vi "DQMH_Event_DialogTest.vi"() -> ()   [LabVIEW 2016]
panel:
  in  "EventData":T1={"ModuleName"="TestStation.lvlib", "EventType"=enum."Request", "AddButtonInAPITester"=FALSE, "EventName"="MyRequest", "EventDescription"="Some Description"}
  out "Numeric Control":i32=3
  out "Array":string[][](array[string])=[["Module", "Ring", ""], ["Event Type", "Ring", "Request,Broadcast,Request and Wait for Reply,Round Trip (Request and Wait for Reply + Broadcast)"], ["Add Tester Button", "Boolean", ""], ["Enqueue Message VI", "RadioButtonsControl", ""], ["Existing Request", "Ring", ""], ["Custom Enqueue VI", "Path", ""], ["Broadcast Argument Source", "RadioButtonsControl", ""], ["Event Name", "String", ""], ["Round Trip (Broadcast)", "String", ""], ["Event Description", "String", ""], ["OK", "Boolean", ""], ["Cancel", "Boolean", ""], ["Help", "Boolean", ""], ["Round Trip (Request)", "String", ""], ["Step 6", "String", ""], ["Context Help", "Ring", "Request Event:\nAn event generated by a caller that the module is registered to receive. Typically a request event is a request for the module to \"Do something\".,Broadcast Event:\nAn event generated by the module to let any external code that is registered  to receive the event know that \"Something happened\".,Request and Wait for Reply:\nA request event where the event generator waits for the module to process the request and return the request processing results. This provides synchronous request and reply functionality.,Round Trip:\nA request and wait for reply event and a broadcast event where the reply payload data type is the same as the broadcast argument.,"]]
  out "NI.LV.Dialog Found":bool=TRUE
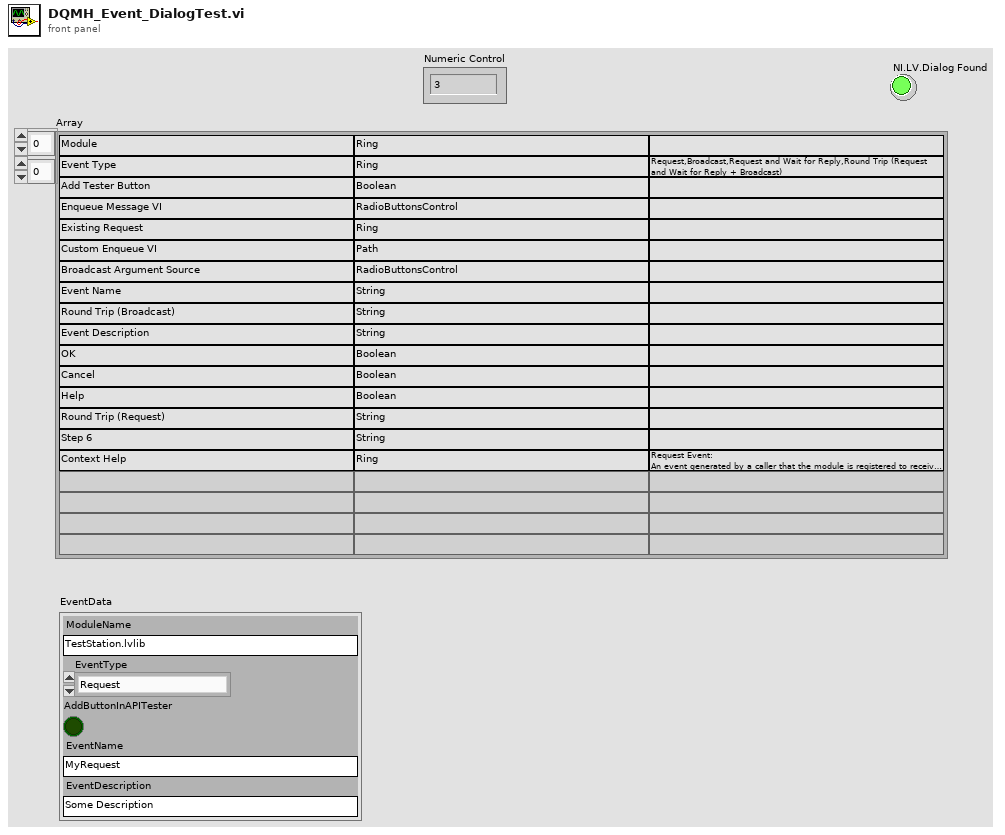
[diagram p1: front panel]
types:
  T1 = cluster{"ModuleName":string, "EventType":enum16{"Request", "Broadcast", "Request and Wait for Reply", "Round Trip"}, "AddButtonInAPITester":bool, "EventName":string, "EventDescription":string}
  T2 = enum32{"Bad", "Idle", "Run top level", "Running"}
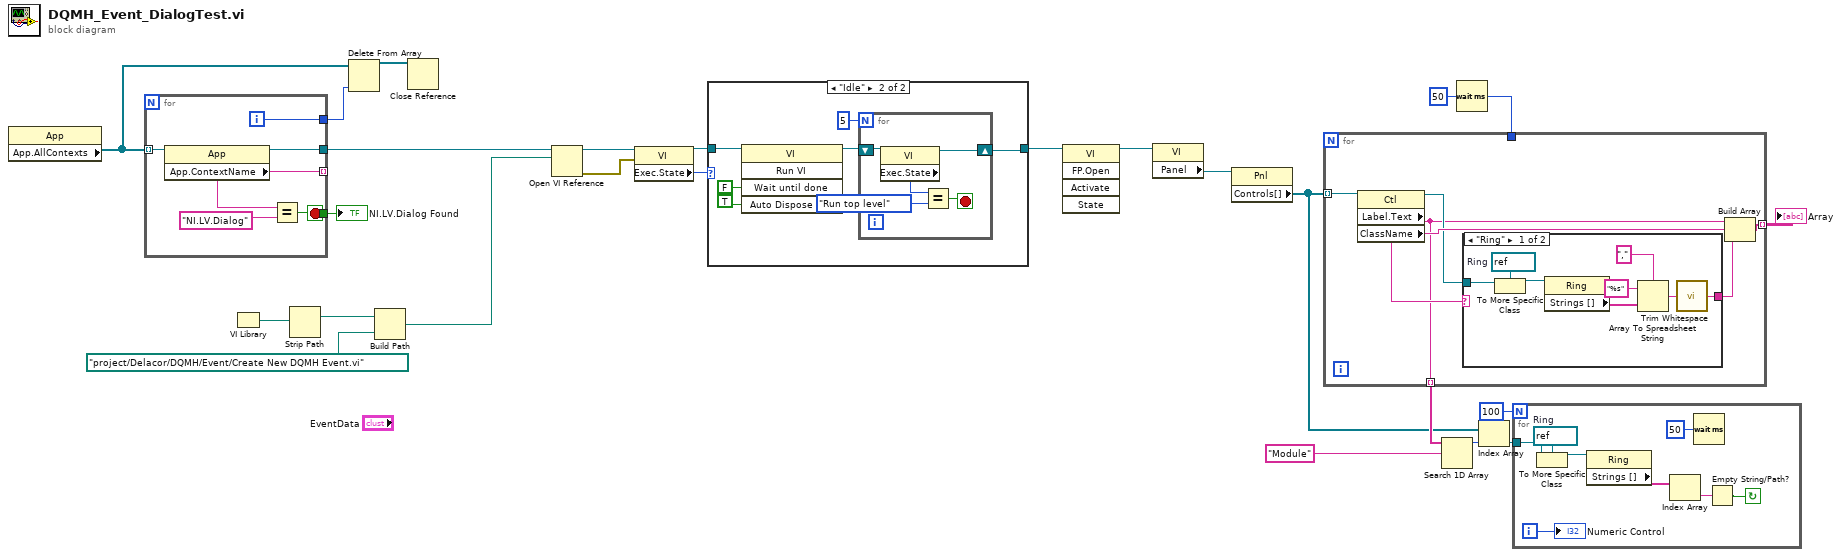
[diagram p0: block diagram]
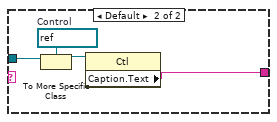
[diagram p2: hidden frame]
diagram:
  n1 = property class="App"() -> ("App.AllContexts"=w24:refnum<vi>[])  [unwired: 2 in, 2 out]
  n2 = for {
    tunnel: w24 -> [w31] mode=indexing
    tunnel: [w29] -> _ mode=indexing
    tunnel: [w28] -> w25
    tunnel: [w27] -> w23
    tunnel: [w26] -> w21
    i -> [w27]
    stop <- w28 stop-if-true
    n3 = property class="App"(reference=w31) -> (reference out=w26:refnum<vi>, "App.ContextName"=w29:string)  [unwired: 1 in, 1 out]
    n4 = Equal?(x=w29, y="NI.LV.Dialog" ("App.ContextName")) -> (x = y?=w28:bool)
  }
  "NI.LV.Dialog Found" <- w25
  n5 = VI Library() -> (path=w20:path)
  n6 = Strip Path(path=w20) -> (stripped path=w19:path)  [unwired: 1 out]
  n7 = Delete From Array(array=w24, index=w23) -> (array with subset deleted=w22:refnum<vi>[])  [unwired: 1 in, 1 out]
  n8 = Build Path(base path=w19, name or relative path=path "project/Delacor/DQMH/Event/Create New DQMH Event.vi") -> (appended path=w17:path)
  n9 = Close Reference(reference=w22) -> ()  [unwired: 1 in, 1 out]
  n10 = Open VI Reference(application reference (local)=w21, vi path=w17) -> (vi reference=w16:refnum<vi>, error out=w15:errorcluster)  [unwired: 4 in]
  n11 = property class="VI"(reference=w16, error in=w15) -> (reference out=w13:refnum<vi>, "Exec.State"=w14:T2)  [unwired: 1 out]
  n12 = case shown="\"Idle\"" w14 {
    tunnel: w13 -> [w32 w38]
    tunnel: [w32 w33] -> w11
    frame "Bad", Default {
    }
    frame "Idle" {
      n13 = invoke class="VI" method="Run VI"(reference=w38, "Wait until done"=FALSE ("Wait Until Done"), "Auto Dispose Ref"=TRUE ("Wait Until Done")) -> (reference out=w35:refnum<vi>)  [unwired: 2 in, 4 out]
      n14 = for {
        N: 5 -> [_]
        shift-right: [w39] -> w33
        shift-left: w35 -> [w43]
        stop <- w40 stop-if-true
        n15 = property class="VI"(reference=w43) -> (reference out=w39:refnum<vi>, "Exec.State"=w42:T2)  [unwired: 1 in, 1 out]
        n16 = Equal?(x=w42, y=T2."Run top level") -> (x = y?=w40:bool)
      }
    }
  }
  n17 = invoke class="VI" method="FP.Open"(reference=w11) -> (reference out=w10:refnum<vi>)  [unwired: 4 in, 4 out]
  n18 = property class="VI"(reference=w10) -> ("Panel"=w12:refnum<vi>)  [unwired: 1 in, 2 out]
  n19 = property class="Pnl"(reference=w12) -> ("Controls[]"=w5:refnum<vi>[])  [unwired: 1 in, 2 out]
  n20 = Wait (ms)(milliseconds to wait=u32 50) -> (millisecond timer value=w1:u32)
  n21 = for {
    tunnel: w5 -> [w49] mode=indexing
    tunnel: [w48] -> w9 mode=indexing
    tunnel: [w44] -> w8 mode=indexing
    tunnel: w1 -> [_]
    n22 = property class="Ctl"(reference=w49) -> (reference out=w46:refnum<vi>, "Label.Text"=w44:string, "ClassName"=w47:string)  [unwired: 1 in, 1 out]
    n23 = case shown="\"Ring\"" w47 {
      tunnel: w46 -> [w57 w61]
      tunnel: [w50 w58] -> w45
      frame "Ring" {
        w56 = refnum<vi> refnum  # Ring
        n24 = To More Specific Class(target class=w56, reference=w57) -> (specific class reference=w55:refnum<vi>)  [unwired: 1 in, 1 out]
        n25 = property class="Ring"(reference=w55) -> ("Strings []"=w54:string[])  [unwired: 1 in, 2 out]
        n26 = Array To Spreadsheet String(delimiter (Tab)=",", array=w54, 3:"%s" ("format string")) -> (spreadsheet string=w51:string)
        n27 = call <vilib>:"Trim Whitespace.vi"("string"=w51) -> ("trimmed string"=w50:string)  [unwired: 1 in]
      }
      frame Default {
        w60 = refnum<vi> refnum  # Control
        n28 = To More Specific Class(target class=w60, reference=w61) -> (specific class reference=w59:refnum<vi>)  [unwired: 1 in, 1 out]
        n29 = property class="Ctl"(reference=w59) -> ("Caption.Text"=w58:string)  [unwired: 1 in, 2 out]
      }
    }
    n30 = Build Array(w44, w47, w45) -> (w48:string[])
  }
  "Array" <- w9
  n31 = Search 1D Array(1D array=w8, element="Module" ("String")) -> (index of element=w4:i32)  [unwired: 1 in]
  n32 = Index Array(array=w5, index=w4) -> (element=w3:refnum<vi>)
  n33 = for {
    N: 100 -> [_]
    tunnel: w3 -> [w67]
    i -> [w65]
    stop <- w62 continue-if-true
    w68 = refnum<vi> refnum  # Ring
    n34 = To More Specific Class(target class=w68, reference=w67) -> (specific class reference=w69:refnum<vi>)  [unwired: 1 in, 1 out]
    n35 = property class="Ring"(reference=w69) -> ("Strings []"=w64:string[])  [unwired: 1 in, 2 out]
    n36 = Index Array(array=w64) -> (element=w63:string)  [unwired: 1 in]
    n37 = Wait (ms)(milliseconds to wait=u32 50) -> ()  [unwired: 1 out]
    n38 = Empty String/Path?(string/path=w63) -> (empty?=w62:bool)
    "Numeric Control" <- w65
  }
